vi "_PC_NS_Wfm_Destory.vi"(5 "wfm stop bool":refnum<k21>, 8 "error in (no error)":errorcluster, 11 "writer name In":refnum<k21>) -> (0 "error out":errorcluster)   [LabVIEW 2018]
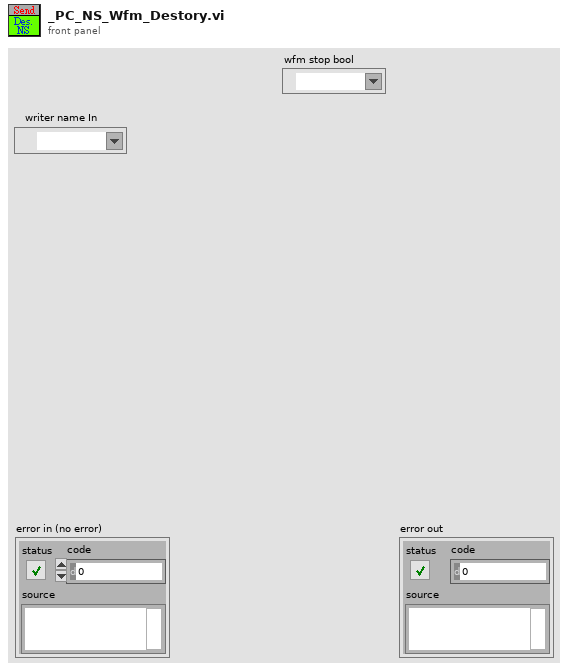
[diagram p1: front panel]
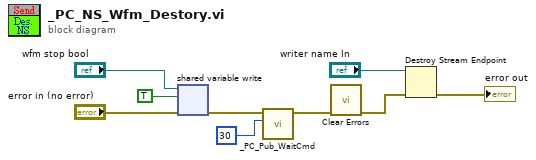
[diagram p0: block diagram]
diagram:
  n1 = shared-variable-write("wfm stop bool", "error in (no error)", TRUE ("data in")) -> (w1:errorcluster)  [unwired: 1 out]
  n2 = call "_PC_Pub_WaitCmd.vi"("milliseconds to wait"=u32 30, "error in (no error)"=w1) -> ("error out"=w5:errorcluster)  [unwired: 9 in]
  n3 = call <vilib>:"Clear Errors.vi"("error in (no error)"=w5) -> ("error out"=w8:errorcluster)  [unwired: 5 in, 1 out]
  n4 = Destroy Stream Endpoint(8:w8, 11:"writer name In") -> (0:→"error out":errorcluster)
